vi "Move_Motor_modified.vi"(0 "VISA Refnum in":refnum<visa-resource-name>, 5 "Motor ID (0)":u8, 7 "Goal Position (bit)":dbl=150.0, 9 "Goal Speed (RPM)":dbl, 11 "error in (no error)":errorcluster) -> (4 "VISA Refnum out":refnum<visa-resource-name>, 15 "error out":errorcluster)   [LabVIEW 2015]
uses:
  <instrlib>/Dynamixel Motor/Dynamixel Motor.lvlib
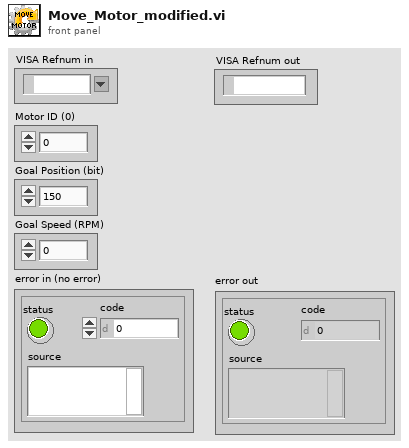
[diagram p1: front panel]
types:
  T1 = enum16{"big-endian, network order", "native, host order", "little-endian"}
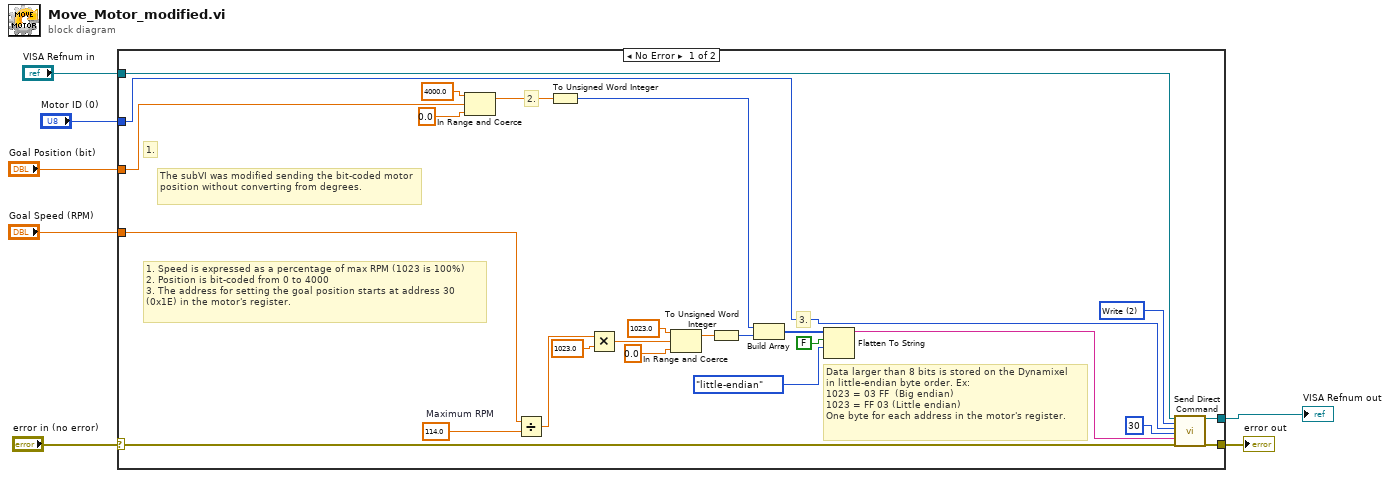
[diagram p0: block diagram]
diagram:
  n1 = case shown="No Error" "error in (no error)" {
    selector: "error in (no error)" -> [w12 w34]
    tunnel: "VISA Refnum in" -> [w31 w33]
    tunnel: [w30 w33] -> w1
    tunnel: [w29 w34] -> w7
    tunnel: "Motor ID (0)" -> [w28 _]
    tunnel: "Goal Position (bit)" -> [w8 _]
    tunnel: "Goal Speed (RPM)" -> [w23 _]
    frame No Error {
      w20 = 114.0  # Maximum RPM
      w32 = u16 2 items=["Ping", "Read", "Write", "Registered Write", "Action", "Reset", "Sync Write"] ("Select Action")
      # "The subVI was modified sending the bit-coded motor position without converting from degrees."
      # "3."
      # "2."
      # "1."
      # "Data larger than 8 bits is stored on the Dynamixel \nin little-endian byte order. Ex:\n1023 = 03 FF  (Big endian)\n1023 = FF 03 (Little endian)\nOne byte for each address in the motor's register."
      # "1. Speed is expressed as a percentage of max RPM (1023 is 100%)\n2. Position is bit-coded from 0 to 4000\n3. The address for setting the goal position starts at address 30\n(0x1E) in the motor's register."
      n2 = In Range and Coerce(upper limit=4000.0, x=w8, lower limit=0.0) -> (coerced(x)=w9:dbl)  [unwired: 1 out]
      n3 = Divide(x=w23, y=w20) -> (x/y=w22:dbl)
      n4 = To Unsigned Word Integer(number=w9) -> (unsigned 16bit integer=w17:u16)
      n5 = Multiply(x=w22, y=1023.0 ("upper limit")) -> (x*y=w26:dbl)
      n6 = In Range and Coerce(upper limit=1023.0, x=w26, lower limit=0.0) -> (coerced(x)=w14:dbl)  [unwired: 1 out]
      n7 = To Unsigned Word Integer(number=w14) -> (unsigned 16bit integer=w16:u16)
      n8 = Build Array(w17, w16) -> (w15:u16[])
      n9 = Flatten To String(anything=w15, prepend array or string size? (T)=FALSE, byte order (0:big-endian, network order)=T1."little-endian") -> (data string=w13:string)  [unwired: 1 in, 2 out]
      n10 = call <instrlib>:"Send Direct Command.vi"("VISA resource name"=w31, "Select Action"=w32, "Motor ID (0)"=w28, "Address"=u8 30, "Parameters"=w13, "Error in (no error)"=w12) -> ("VISA resource name out"=w30:refnum<visa-resource-name>, "Error out"=w29:errorcluster)  [unwired: 11 in, 1 out]
    }
    frame Error {
    }
  }
  "error out" <- w7
  "VISA Refnum out" <- w1
